vi "Command and query iterating.vi"(8 "error in (no error)":errorcluster, 9 "delay before read (ms)":u32=10, 10 "Command String":string="?VW", 11 "Serial_comms in":refnum<class "Serial_comms.lvclass">) -> (0 "error out":errorcluster, 1 "output cluster":T1, 2 "Response":string, 3 "Serial_comms out":refnum<class "Serial_comms.lvclass">)   [LabVIEW 2020, in "Serial_comms.lvlib" / "Serial_comms.lvclass"]
uses:
  Serial_comms.lvclass
panel:
  out "bytes read":u32
  out "return count":u32
  out "Bytes at port loop itr":i32
  out "Read bytes loop itr":i32
  out "Bytes at port failed":bool
  out "Read bytes failed":bool
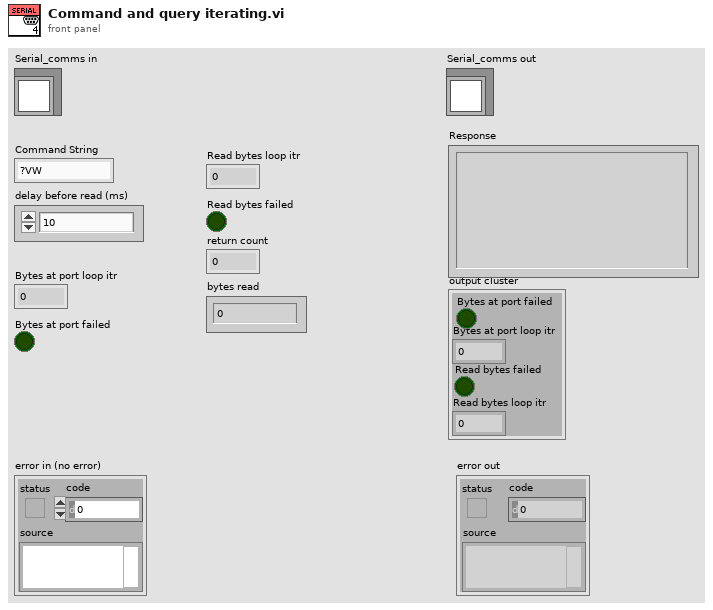
[diagram p1: front panel]
types:
  T1 = cluster{"Bytes at port failed":bool, "Bytes at port loop itr":i32, "Read bytes failed":bool, "Read bytes loop itr":i32}
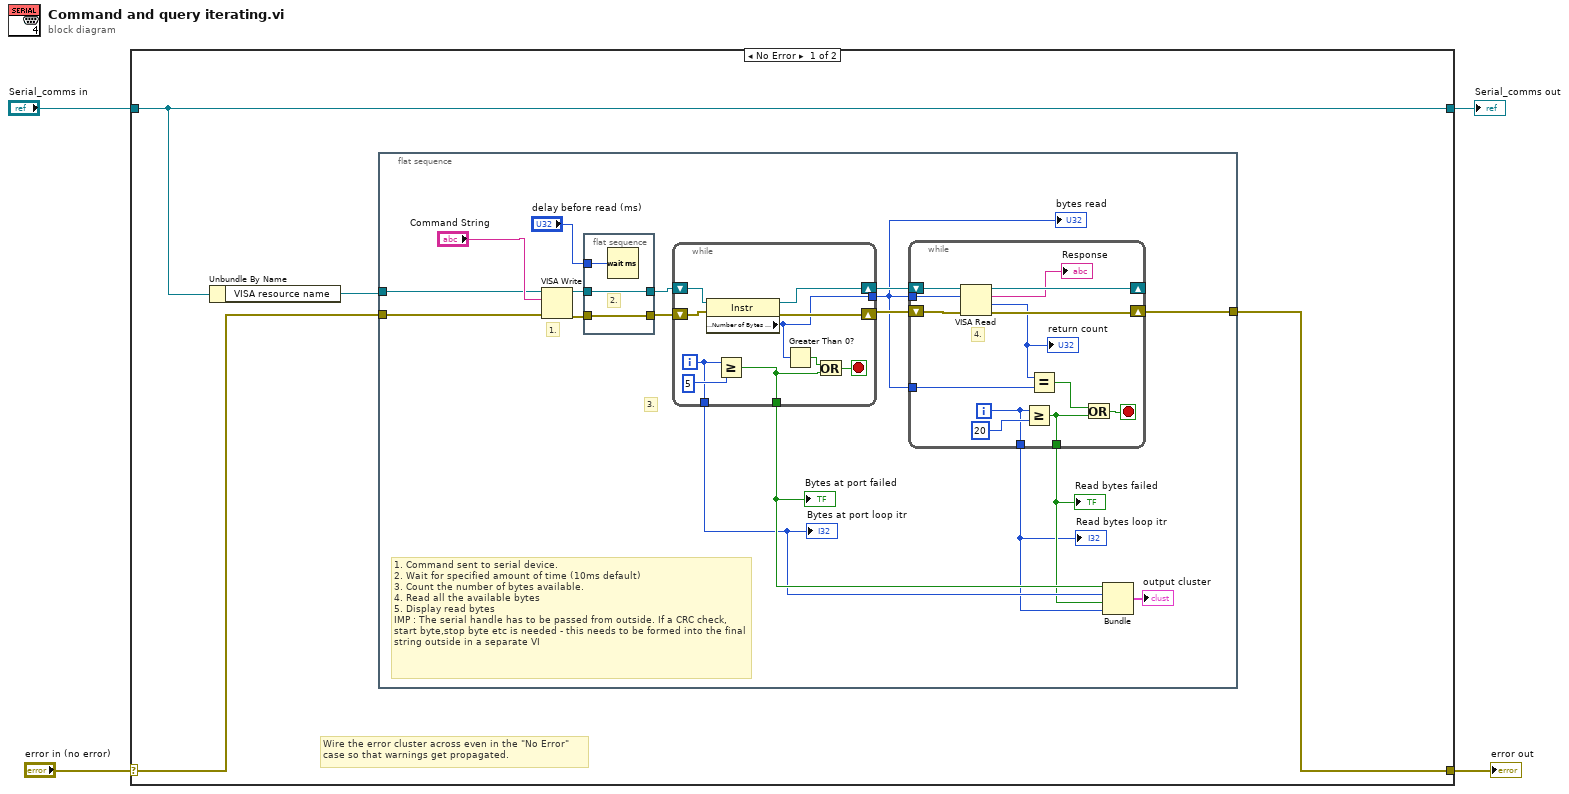
[diagram p0: block diagram]
diagram:
  n1 = case shown="No Error" "error in (no error)" {
    selector: "error in (no error)" -> [w6 w53]
    tunnel: [w5 w53] -> w3
    tunnel: [w8 w52] -> w1
    tunnel: "Serial_comms in" -> [w8 w52]
    frame No Error {
      # "Wire the error cluster across even in the \"No Error\"\ncase so that warnings get propagated."
      n2 = Unbundle By Name(w8) -> ("VISA resource name"=w7:refnum<visa-resource-name>)
      n3 = flat-sequence {
        tunnel: w7 -> [w11]
        tunnel: w6 -> [w10]
        tunnel: [w9] -> w5
        frame #0 {
          # "3."
          # "1."
          # "1. Command sent to serial device.\n2. Wait for specified amount of time (10ms default)\n3. Count the number of bytes available.\n4. Read all the available bytes\n5. Display read bytes\nIMP : The serial handle has to be passed from outside. If a CRC check, start byte,stop byte etc is needed - this needs to be formed into the final string outside in a separate VI"
          n4 = VISA Write(VISA resource name=w11, write buffer="Command String", error in (no error)=w10) -> (VISA resource name out=w23:refnum<visa-resource-name>, error out=w21:errorcluster)  [unwired: 1 out]
          n5 = flat-sequence {
            tunnel: w21 -> [w50]
            tunnel: [w50] -> w22
            tunnel: w23 -> [w49]
            tunnel: [w49] -> w24
            tunnel: "delay before read (ms)" -> [w51]
            frame #0 {
              # "2."
              n6 = Wait (ms)(milliseconds to wait=w51) -> ()  [unwired: 1 out]
            }
          }
          n7 = while {
            tunnel: [w44] -> w17
            shift-right: [w45] -> w18
            shift-left: w24 -> [w48]
            shift-right: [w46] -> w19
            shift-left: w22 -> [w47]
            tunnel: [w40] -> w15
            tunnel: [w39] -> w16
            i -> [w40]
            stop <- w41 stop-if-true
            n8 = property class="Instr"(reference=w48, error in=w47) -> (reference out=w45:refnum<visa-resource-name>, error out=w46:errorcluster, "Serial Settings:Number of Bytes at Serial Port"=w44:u32)
            n9 = Greater Or Equal?(x=w40, y=5) -> (x >= y?=w39:bool)
            n10 = Greater Than 0?(x=w44) -> (x > 0?=w42:bool)
            n11 = Or(x=w42, y=w39) -> (x .or. y?=w41:bool)
          }
          "bytes read" <- w17
          "Bytes at port loop itr" <- w15
          "Bytes at port failed" <- w16
          n12 = while {
            tunnel: w17 -> [w35]
            shift-right: [w38] -> w9
            shift-left: w19 -> [w34]
            shift-right: [w37] -> _
            shift-left: w18 -> [w33]
            tunnel: w17 -> [w31]
            tunnel: [w27] -> w13
            tunnel: [w26] -> w14
            i -> [w27]
            stop <- w28 stop-if-true
            # "4."
            n13 = VISA Read(VISA resource name=w33, byte count=w35, error in (no error)=w34) -> (VISA resource name out=w37:refnum<visa-resource-name>, read buffer=→"Response":string, return count=w32:u32, error out=w38:errorcluster)
            "return count" <- w32
            n14 = Greater Or Equal?(x=w27, y=20) -> (x >= y?=w26:bool)
            n15 = Equal?(x=w32, y=w31) -> (x = y?=w29:bool)
            n16 = Or(x=w29, y=w26) -> (x .or. y?=w28:bool)
          }
          "Read bytes loop itr" <- w13
          "Read bytes failed" <- w14
          n17 = Bundle(w16, w15, w14, w13) -> (→"output cluster":cluster{bool, i32, bool, i32})  [unwired: 1 in]
        }
      }
    }
    frame Error {
    }
  }
  "error out" <- w3
  "Serial_comms out" <- w1
